vi "Exponential Smoothing.vi"() -> ()   [LabVIEW 2023]
doc: "This example shows how to perform exponential average on a univariate time series with the TSA Exponential Average VI.\n\n<b>Instructions:</b>\n1) Run this VI.\n2) Try different settings for exponential smoothing and observe the results."
uses:
  <vilib>/addons/Time Series Analysis/Utilities.llb/TSA Data.ctl
  <vilib>/addons/Time Series Analysis/Series Preprocess.llb/TSA Exponential Average (Array).vi
  <vilib>/addons/_Advanced Signal Processing/NI_AdvSigProcTSA.lvlib
panel:
  in  "stop":bool
  in  "Season type":u16(ring)=1 items=["Multiplicative", "Additive"]
  in  "Season period":i32=4
  in  "Exponential factors 3":cluster{"Level":dbl, "Trend":dbl, "Season":dbl}={"Level"=0.30000000000000016, "Trend"=0.5000000000000001, "Season"=0.8} {"Season" step=0.1; "Trend" step=0.1; "Level" step=0.1}
  in  "Exponential factors 2":cluster{"Level":dbl, "Trend":dbl, "Season":dbl}={"Level"=0.30000000000000016, "Trend"=0.5000000000000001, "Season"=0.9} {"Trend" step=0.1; "Level" step=0.1}
  in  "Exponential factors 1":cluster{"Level":dbl, "Trend":dbl, "Season":dbl}={"Level"=0.30000000000000016, "Trend"=0.9, "Season"=0.9} {"Level" step=0.1}
  out "Period Product Sales":dbl[][](graph)
  # "Overview: Shows how to perform exponential average on a univariate time series with the TSA Exponential Average VI.\nRequirements: LabVIEW Full Development System, Advanced Signal Processing Toolkit\nInstructions: \n1. Run this VI.\n2. Try different settings for exponential smoothing and observe the results.\n3. Click Stop to stop the VI."
  # "Single Exp Smoothing"
  # "Double Exp Smoothing"
  # "Triple Exp Smoothing"
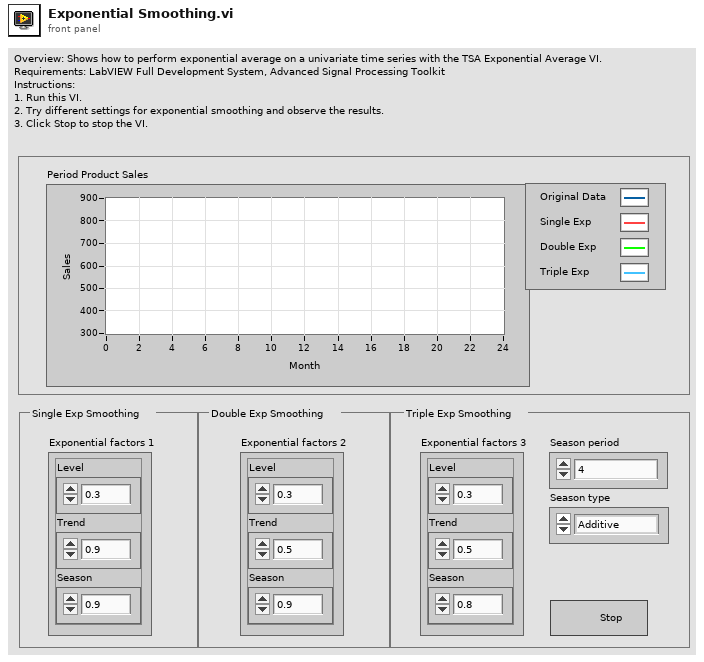
[diagram p1: front panel]
types:
  T1 = typedef "NI_AdvSigProcTSA.lvlib/TSA Data.ctl" = u16
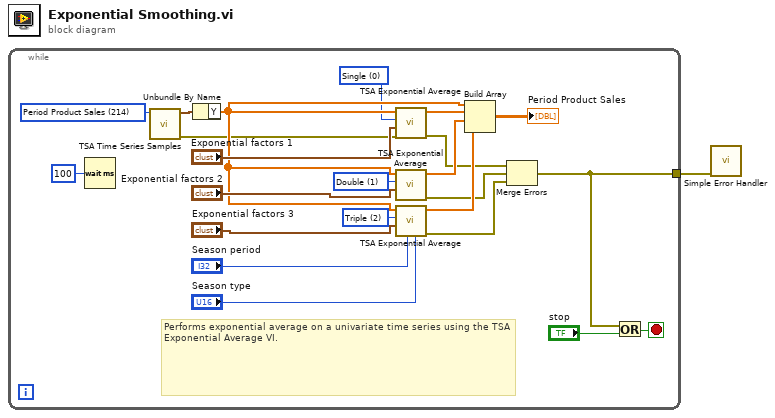
[diagram p0: block diagram]
diagram:
  n1 = while {
    tunnel: [w3] -> w1
    stop <- w6 stop-if-true
    w4 = T1 214 items=["Kobe Earthquake"=201, "EEG"=210, "Bearing Vibration (simulated)"=211, "Period Product Sales"=214, "Beam Vibration (nonlinear)"=217, "Beam Vibration (linear)"=218, "Signal With Echo"=219, "Engine Knocking"=220, "Power Line"=221, "-"=200, "Beam Deflections (multivariate)"=207, "Structure Vibration (multivariate)"=208, "Human MEG (multivariate)"=222] ("data")
    w12 = u16 2 items=["Single", "Double", "Triple"] ("exponential type")
    w13 = u16 1 items=["Single", "Double", "Triple"] ("exponential type")
    w14 = u16 0 items=["Single", "Double", "Triple"] ("exponential type")
    # "Performs exponential average on a univariate time series using the TSA Exponential Average VI."
    n2 = Wait (ms)(milliseconds to wait=u32 100 ("millisecond multiple")) -> ()  [unwired: 1 out]
    n3 = call <vilib>:"TSA Time Series Samples.vi"("data"=w4) -> ("error out"=w2:errorcluster, "univariate time series"=w16:waveform(dbl))  [unwired: 1 in, 8 out]
    n4 = Unbundle By Name(w16) -> ("Y"=w15:dbl[])
    n5 = call-poly <vilib>:"TSA Exponential Average.vi"("error in (no error)"=w2, "exponential factors"="Exponential factors 1", "exponential type"=w14, "Xt"=w15) -> ("error out"=w10:errorcluster, "Xt averaged"=w24:dbl[])  [unwired: 6 out]
    n6 = call-poly <vilib>:"TSA Exponential Average.vi"("exponential factors"="Exponential factors 2", "exponential type"=w13, "Xt"=w15) -> ("error out"=w9:errorcluster, "Xt averaged"=w22:dbl[])  [unwired: 1 in, 6 out]
    n7 = call-poly <vilib>:"TSA Exponential Average.vi"("season type"="Season type", "season period"="Season period", "exponential factors"="Exponential factors 3", "exponential type"=w12, "Xt"=w15) -> ("error out"=w8:errorcluster, "Xt averaged"=w21:dbl[])  [unwired: 1 in, 4 out]
    n8 = Build Array(w15, w24, w22, w21) -> (→"Period Product Sales":dbl[][])
    n9 = Merge Errors(w10, w9, w8) -> (w3:errorcluster)
    n10 = Or(x=w3, y="stop") -> (x .or. y?=w6:bool)
  }
  n11 = call <vilib>:"Simple Error Handler.vi"("error in (no error)"=w1) -> ()  [unwired: 1 in, 8 out]
